vi "Build Node URL.vi"(7 "Node Name":string, 8 "error in (no error)":errorcluster, 10 "Path":string, 11 "VolatusAPI in":refnum<class "VolatusAPI.lvclass">) -> (0 "error out":errorcluster, 2 "Request URL":string, 3 "VolatusAPI out":refnum<class "VolatusAPI.lvclass">)   [LabVIEW 2020, in "Volatus.lvlib" / "VolatusAPI.lvclass"]
uses:
  VolatusAPI.lvclass
  VolatusAPI.lvclass/VolatusAPI.ctl
  VolatusConfig/Node/Node Config.lvclass
  VolatusConfig/Cluster/Cluster Config.lvclass
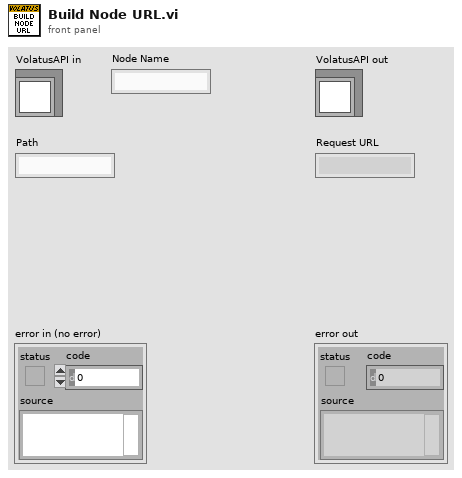
[diagram p1: front panel]
types:
  T1 = typedef "TcpClientList.lvlib/Data.ctl" = cluster{"clients":T2[]}
  T2 = typedef "TcpClientInfo.lvlib/Data.ctl" = cluster{"node_id":u32, "node_name":string, "app_version":string, "config_version":string, "config_hash":string, "node_alias":string, "address":string}
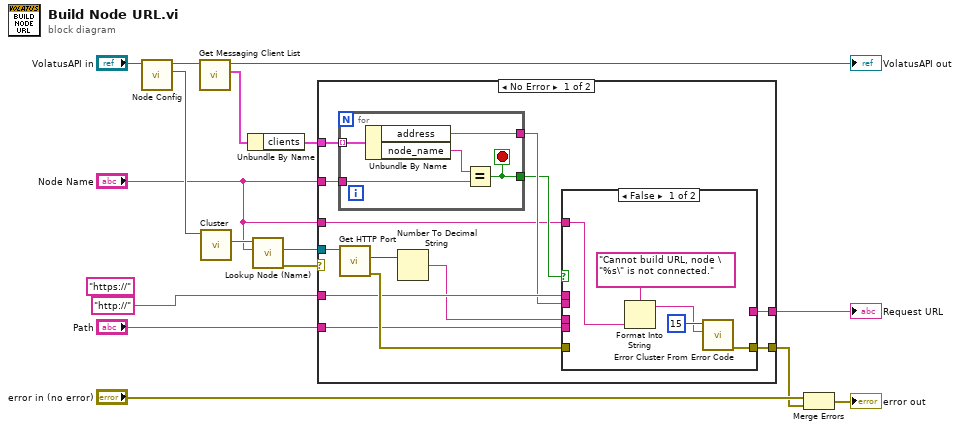
[diagram p0: block diagram]
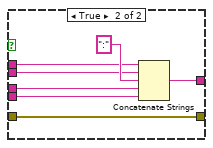
[diagram p2: hidden frame]
diagram:
  (unwired) "https://"
  n1 = call "Node Config.vi"("VolatusAPI in"="VolatusAPI in") -> ("Node Config"=w6:refnum<class "Node Config.lvclass">, "VolatusAPI out"=w7:refnum<class "VolatusAPI.lvclass">)  [unwired: 9 in]
  n2 = call "Get Messaging Client List.vi"("VolatusAPI in"=w7) -> ("Client List"=w9:T1, "VolatusAPI out"=→"VolatusAPI out":refnum<class "VolatusAPI.lvclass">)  [unwired: 8 in, 1 out]
  n3 = call "Cluster.vi"("Node in"=w6) -> ("Cluster"=w5:refnum<class "Cluster Config.lvclass">)  [unwired: 8 in, 2 out]
  n4 = Unbundle By Name(w9) -> ("clients"=w8:T2[])
  n5 = call "Lookup Node (Name).vi"("Node Name"="Node Name", "Cluster in"=w5) -> ("error out"=w4:errorcluster, "Node"=w3:refnum<class "Node Config.lvclass">)  [unwired: 7 in, 1 out]
  n6 = case shown="No Error" w4 {
    selector: w4 -> [_ w47]
    tunnel: "Path" -> [w28 _]
    tunnel: "http://" -> [w27 _]
    tunnel: [w23 _] -> w12
    tunnel: w8 -> [w26 _]
    tunnel: "Node Name" -> [w25 _]
    tunnel: w3 -> [w24 _]
    tunnel: [w17 w47] -> w2
    tunnel: "Node Name" -> [w18 _]
    frame No Error {
      n7 = for {
        tunnel: w26 -> [w46] mode=indexing
        tunnel: w25 -> [w45]
        tunnel: [w43] -> w20
        tunnel: [w42] -> w19
        stop <- w42 stop-if-true
        n8 = Unbundle By Name(w46) -> ("address"=w43:string, "node_name"=w44:string)
        n9 = Equal?(x=w44, y=w45) -> (x = y?=w42:bool)
      }
      n10 = call "Get HTTP Port.vi"("Node Config in"=w24) -> ("error out"=w29:errorcluster, "HTTP Port"=w22:u16)  [unwired: 8 in, 1 out]
      n11 = Number To Decimal String(number=w22) -> (decimal integer string=w21:string)  [unwired: 1 in]
      n12 = case shown="False" w19 {
        tunnel: w28 -> [_ w40]
        tunnel: w27 -> [_ w39]
        tunnel: [_ w38] -> w23
        tunnel: w21 -> [_ w37]
        tunnel: w20 -> [_ w36]
        tunnel: w18 -> [w31 _]
        tunnel: [w32 w35] -> w17
        tunnel: w29 -> [_ w35]
        frame False {
          n13 = Format Into String(format string="Cannot build URL, node \"%s\" is not connected.", w31) -> (resulting string=w33:string)  [unwired: 2 in, 1 out]
          n14 = call <vilib>:"Error Cluster From Error Code.vi"("error message (\"\")"=w33, "error code (0)"=15) -> ("error out"=w32:errorcluster)  [unwired: 7 in]
        }
        frame True {
          n15 = Concatenate Strings(w39, w36, ":" ("string"), w37, w40) -> (w38:string)
        }
      }
    }
    frame Error {
    }
  }
  "Request URL" <- w12
  n16 = Merge Errors("error in (no error)", w2) -> (→"error out":errorcluster)
